vi "Create_Reg_Cluster.vi"(9 "Analog mode?":bool, 10 "Double resolution?":bool, 11 "Auto calibrate?":bool) -> (3 "Cluster output":T1)   [LabVIEW 2017, in "GP22_TDC_Arduinoed.lvlib"]
doc: "Creates a cluster of values to set the GP22's internal registers.\nThis subVI uses ACAM's default settings, modified as requested by the user"
uses:
  GP22_TDC_Arduinoed.lvlib
  Public/Globals.vi
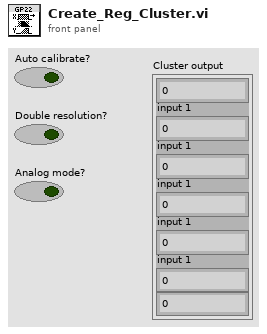
[diagram p1: front panel]
types:
  T1 = cluster{u32, "input 1":u32, "input 1":u32, "input 1":u32, "input 1":u32, "input 1":u32, u32}
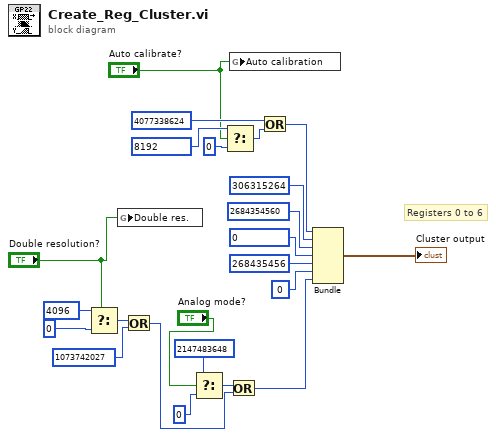
[diagram p0: block diagram]
diagram:
  # "Registers 0 to 6"
  n1 = Select(t=u32 4096 ("input 1"), s="Double resolution?", f=u32 0) -> (s? t:f=w16:u32)
  n2 = global write "Globals.vi" "Double res."("Double resolution?") -> ()
  n3 = Or(x=w16, y=u32 1073742027 ("input 1")) -> (x .or. y?=w3:u32)
  n4 = Select(t=u32 2147483648 ("input 1"), s="Analog mode?", f=u32 0) -> (s? t:f=w6:u32)
  n5 = Select(t=u32 8192 ("input 1"), s="Auto calibrate?", f=u32 0) -> (s? t:f=w11:u32)
  n6 = Or(x=w6, y=w3) -> (x .or. y?=w1:u32)
  n7 = global write "Globals.vi" "Auto calibration"("Auto calibrate?") -> ()
  n8 = Or(x=u32 4077338624 ("input 1"), y=w11) -> (x .or. y?=w17:u32)
  n9 = Bundle(w17, "input 1"=u32 306315264, "input 1"=u32 2684354560, "input 1"=u32 0, "input 1"=u32 268435456, "input 1"=u32 0, w1) -> (→"Cluster output":T1)  [unwired: 1 in]
